vi "addImageToQueue.vi"(8 "error in (no error)":errorcluster, 10 "ImageData":T1, 11 "PixelflySA in":refnum<class "PixelflySA.lvclass">) -> (0 "error out":errorcluster, 3 "PixelflySA out":refnum<class "PixelflySA.lvclass">)   [LabVIEW 2009, in "PixelflySA.lvclass"]
uses:
  PixelflySA.lvclass
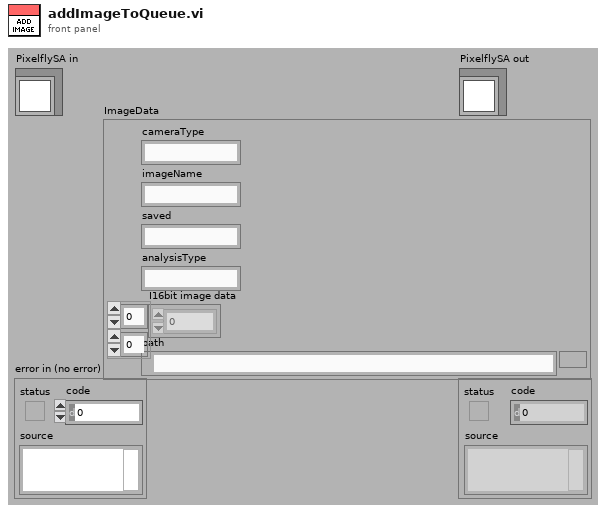
[diagram p1: front panel]
types:
  T1 = cluster{"cameraType":string, "imageName":string, "saved":string, "analysisType":string, "I16bit image data":u16[][], "path":path}
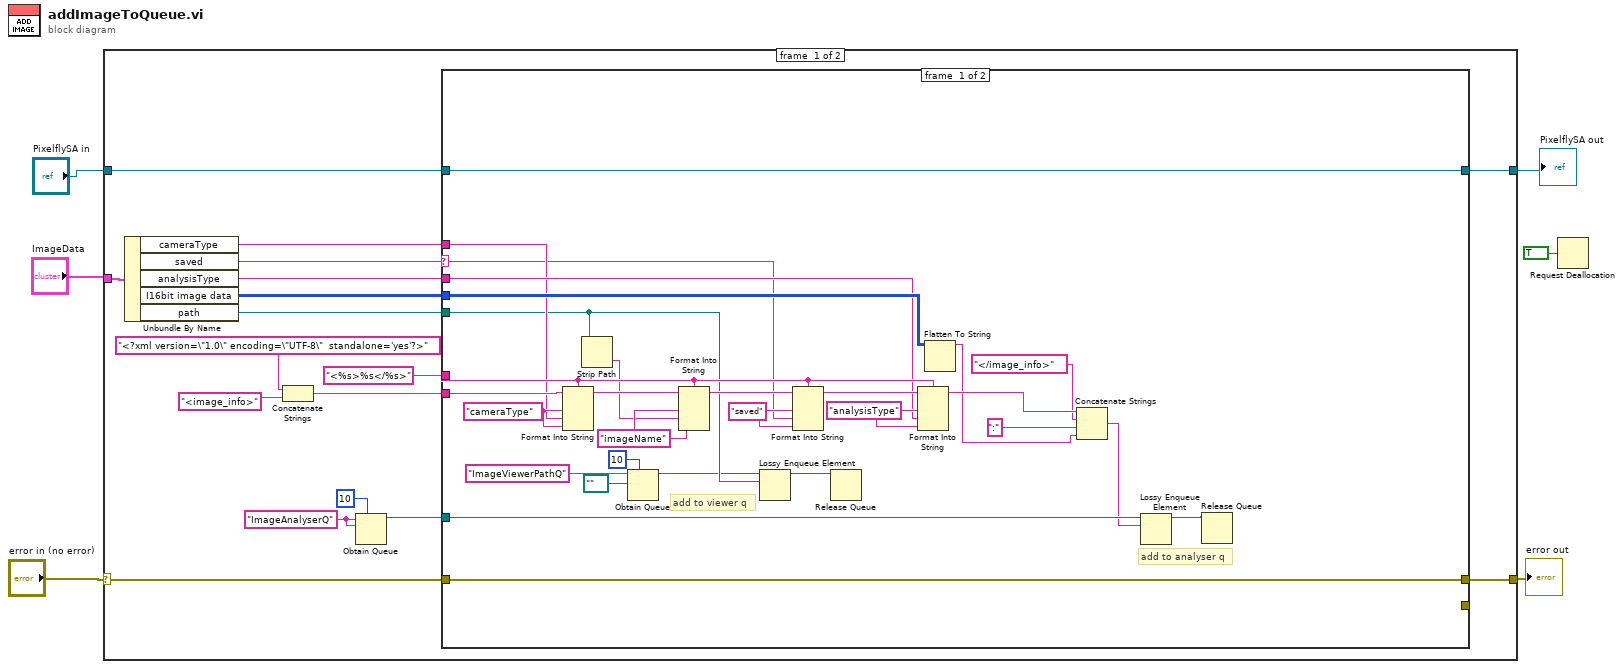
[diagram p0: block diagram]
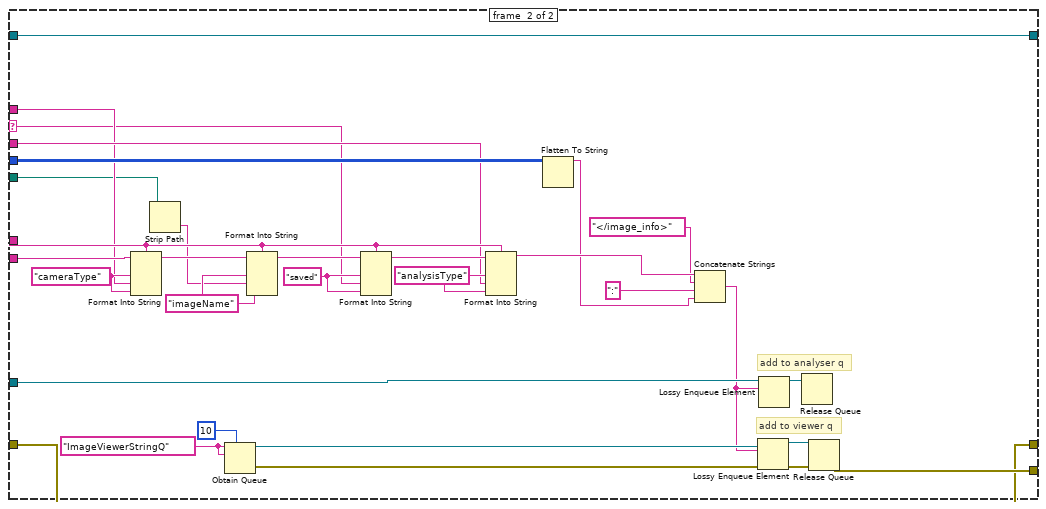
[diagram p2: hidden frame]
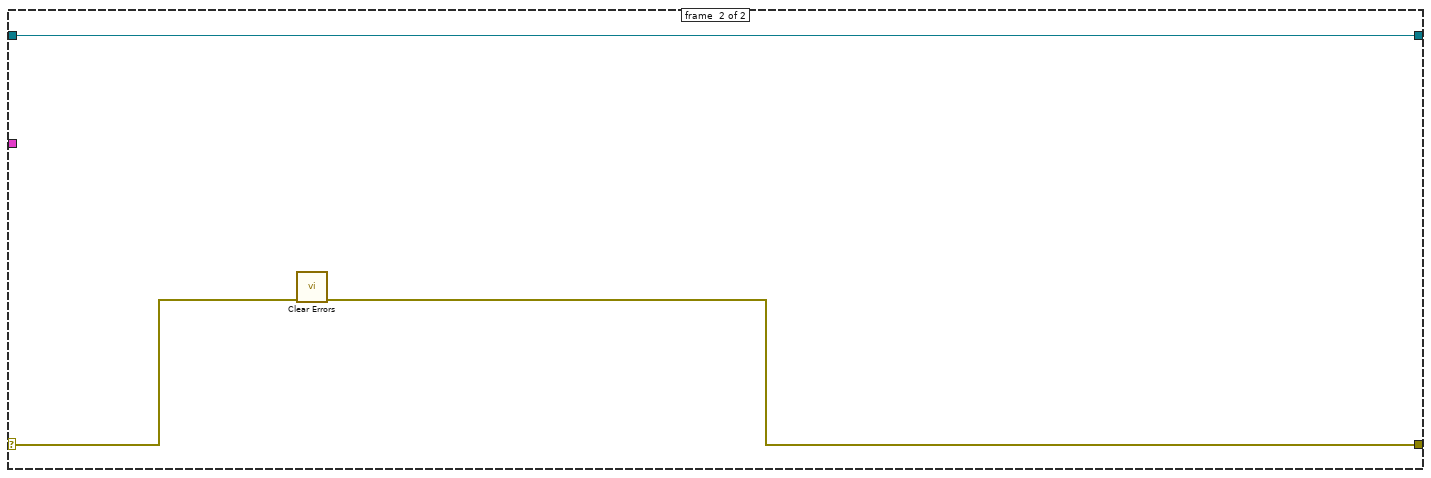
[diagram p3: hidden frame]
diagram:
  n1 = case shown="No Error" "error in (no error)" {
    selector: "error in (no error)" -> [w8 w86]
    tunnel: [w7 w84] -> w3
    tunnel: [w20 w85] -> w4
    tunnel: "PixelflySA in" -> [w22 w85]
    tunnel: "ImageData" -> [w23 _]
    frame #0 {
      w11 = "ImageAnalyserQ"
      n2 = Unbundle By Name(w23) -> ("cameraType"=w19:string, "saved"=w21:string, "analysisType"=w18:string, "I16bit image data"=w17:u16[][], "path"=w16:path)
      n3 = Concatenate Strings("<?xml version=\"1.0\" encoding=\"UTF-8\"  standalone='yes'?>", "<image_info>") -> (w13:string)
      n4 = Obtain Queue(max queue size (-1, unlimited)=10, name (unnamed)=w11, element data type=w11) -> (queue out=w9:refnum<queue>)  [unwired: 2 in, 2 out]
      n5 = case shown="\"false\", Default" w21 {
        selector: w21 -> [w34 w69]
        tunnel: w22 -> [w52 w60]
        tunnel: [w52 w60] -> w20
        tunnel: w19 -> [w35 w70]
        tunnel: w18 -> [w36 w71]
        tunnel: w17 -> [w38 w72]
        tunnel: w16 -> [w33 w68]
        tunnel: w13 -> [w41 w75]
        tunnel: "<%s>%s</%s>" -> [w40 w74]
        tunnel: w9 -> [w32 w67]
        tunnel: w8 -> [w24 w61]
        tunnel: [w24 w61] -> w7
        tunnel: [_ w63] -> _
        frame #0 {
          w49 = "analysisType"
          w47 = "saved"
          w43 = "imageName" ("Key")
          w42 = "cameraType"
          # "add to analyser q"
          # "add to viewer q"
          n6 = Format Into String(format string=w40, initial string=w41, w42, w35, w42) -> (resulting string=w45:string)  [unwired: 1 in, 1 out]
          n7 = Strip Path(path=w33) -> (name=w39:string)  [unwired: 1 out]
          n8 = Obtain Queue(max queue size (-1, unlimited)=10, name (unnamed)="ImageViewerPathQ", element data type=path "") -> (queue out=w27:refnum<queue>)  [unwired: 2 in, 2 out]
          n9 = Format Into String(format string=w40, initial string=w45, w43, w39, w43) -> (resulting string=w46:string)  [unwired: 1 in, 1 out]
          n10 = Lossy Enqueue Element(queue=w27, element=w33) -> (queue out=w26:refnum<queue>)  [unwired: 1 in, 3 out]
          n11 = Format Into String(format string=w40, initial string=w46, w47, w34, w47) -> (resulting string=w50:string)  [unwired: 1 in, 1 out]
          n12 = Release Queue(queue=w26) -> ()  [unwired: 2 in, 3 out]
          n13 = Format Into String(format string=w40, initial string=w50, w49, w36, w49) -> (resulting string=w51:string)  [unwired: 1 in, 1 out]
          n14 = Flatten To String(anything=w38) -> (data string=w37:string)  [unwired: 3 in, 2 out]
          n15 = Concatenate Strings(w51, "</image_info>", ":", w37) -> (w31:string)
          n16 = Lossy Enqueue Element(queue=w32, element=w31) -> (queue out=w25:refnum<queue>)  [unwired: 1 in, 3 out]
          n17 = Release Queue(queue=w25) -> ()  [unwired: 2 in, 3 out]
        }
        frame #1 {
          w65 = "ImageViewerStringQ"
          w81 = "analysisType"
          w80 = "saved"
          w77 = "imageName" ("Key")
          w76 = "cameraType"
          # "add to analyser q"
          # "add to viewer q"
          n18 = Format Into String(format string=w74, initial string=w75, w76, w70, w76) -> (resulting string=w78:string)  [unwired: 1 in, 1 out]
          n19 = Strip Path(path=w68) -> (name=w73:string)  [unwired: 1 out]
          n20 = Obtain Queue(max queue size (-1, unlimited)=10, name (unnamed)=w65, element data type=w65) -> (queue out=w64:refnum<queue>, error out=w62:errorcluster)  [unwired: 2 in, 1 out]
          n21 = Format Into String(format string=w74, initial string=w78, w77, w73, w77) -> (resulting string=w79:string)  [unwired: 1 in, 1 out]
          n22 = Format Into String(format string=w74, initial string=w79, w80, w69, w80) -> (resulting string=w82:string)  [unwired: 1 in, 1 out]
          n23 = Format Into String(format string=w74, initial string=w82, w81, w71, w81) -> (resulting string=w83:string)  [unwired: 1 in, 1 out]
          n24 = Flatten To String(anything=w72) -> (data string=w57:string)  [unwired: 3 in, 2 out]
          n25 = Concatenate Strings(w83, "</image_info>", ":", w57) -> (w56:string)
          n26 = Lossy Enqueue Element(queue=w64, element=w56, error in (no error)=w62) -> (queue out=w54:refnum<queue>, error out=w53:errorcluster)  [unwired: 2 out]
          n27 = Lossy Enqueue Element(queue=w67, element=w56) -> (queue out=w55:refnum<queue>)  [unwired: 1 in, 3 out]
          n28 = Release Queue(queue=w55) -> ()  [unwired: 2 in, 3 out]
          n29 = Release Queue(queue=w54, error in (no error)=w53) -> (error out=w63:errorcluster)  [unwired: 1 in, 2 out]
        }
      }
    }
    frame #1 {
      n30 = call <vilib>:"Clear Errors.vi"("error in (no error)"=w86) -> ("error out"=w84:errorcluster)  [unwired: 6 in]
    }
  }
  "error out" <- w3
  "PixelflySA out" <- w4
  n31 = Request Deallocation(TRUE ("flag")) -> ()
